vi "PID Algorithm.vi"(10 "Piezo Position":dbl, 11 "Feedback Parameters":T1 {"Error Signal Source" items=["External Input", "APD Signal"]}) -> (3 "Signal to Piezo":dbl)   [LabVIEW 2013, in "Feedback.lvlib"]
uses:
  Feedback.lvlib
  Feedback Parameters.ctl
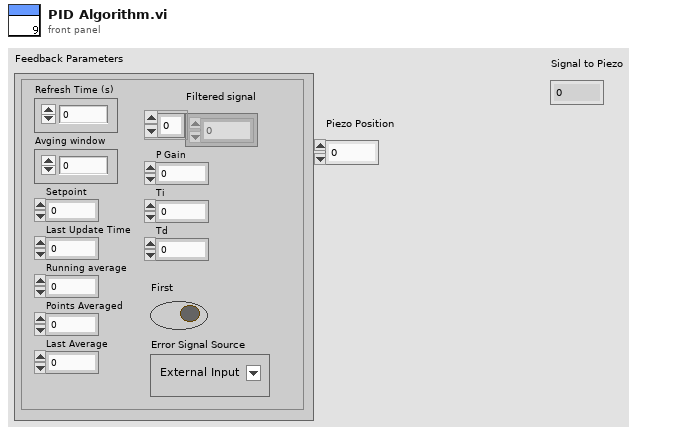
[diagram p1: front panel]
types:
  T1 = typedef "Feedback.lvlib/Feedback Parameters.ctl" = cluster{"Refresh Time (s)":dbl, "P Gain":dbl, "Setpoint":dbl, "Last Update Time":dbl, "Running average":dbl, "Points Averaged":dbl, "Last Average":dbl, "Filtered signal":dbl[], "Avging window":dbl, "Ti":dbl, "Td":dbl, "First":bool, "Error Signal Source":u16}
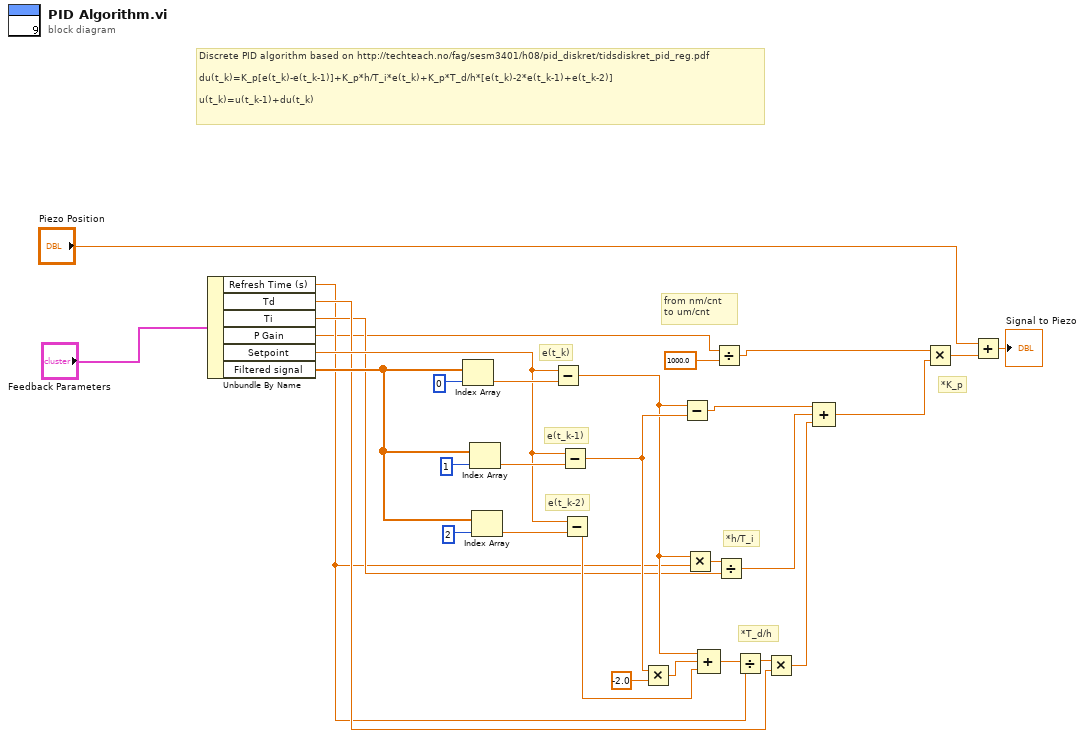
[diagram p0: block diagram]
diagram:
  # "from nm/cnt \nto um/cnt"
  # "*h/T_i"
  # "*T_d/h"
  # "*K_p"
  # "Discrete PID algorithm based on http://techteach.no/fag/sesm3401/h08/pid_diskret/tidsdiskret_pid_reg.pdf\n\ndu(t_k)=K_p[e(t_k)-e(t_k-1)]+K_p*h/T_i*e(t_k)+K_p*T_d/h*[e(t_k)-2*e(t_k-1)+e(t_k-2)]\n\nu(t_k)=u(t_k-1)+du(t_k)"
  # "e(t_k-2)"
  # "e(t_k-1)"
  # "e(t_k)"
  n1 = Unbundle By Name("Feedback Parameters") -> ("Refresh Time (s)"=w4:dbl, "Td"=w6:dbl, "Ti"=w5:dbl, "P Gain"=w1:dbl, "Setpoint"=w19:dbl, "Filtered signal"=w21:dbl[])
  n2 = Index Array(array=w21, index=0) -> (element=w26:dbl)
  n3 = Index Array(array=w21, index=1) -> (element=w24:dbl)
  n4 = Index Array(array=w21, index=2) -> (element=w22:dbl)
  n5 = Subtract(x=w19, y=w26) -> (x-y=w13:dbl)
  n6 = Subtract(x=w19, y=w24) -> (x-y=w14:dbl)
  n7 = Subtract(x=w19, y=w22) -> (x-y=w11:dbl)
  n8 = Multiply(x=w14, y=-2.0) -> (x*y=w12:dbl)
  n9 = Subtract(x=w13, y=w14) -> (x-y=w18:dbl)
  n10 = Multiply(x=w13, y=w4) -> (x*y=w17:dbl)
  n11 = Compound Arithmetic op=ADD(w13, w12, w11) -> (w10:dbl)
  n12 = Divide(x=w1, y=1000.0) -> (x/y=w3:dbl)
  n13 = Divide(x=w17, y=w5) -> (x/y=w16:dbl)
  n14 = Divide(x=w10, y=w4) -> (x/y=w9:dbl)
  n15 = Multiply(x=w9, y=w6) -> (x*y=w8:dbl)
  n16 = Compound Arithmetic op=ADD(w18, w16, w8) -> (w7:dbl)
  n17 = Multiply(x=w3, y=w7) -> (x*y=w20:dbl)
  n18 = Add(x="Piezo Position", y=w20) -> (x+y=→"Signal to Piezo":dbl)
